vi "Configure Channels.vi"(8 "error in":errorcluster, 11 "Thermometer DAQmx RTD Cont CFG in":refnum<class "Thermometer DAQmx RTD Cont CFG.lvclass">) -> (0 "error out":errorcluster, 3 "Thermometer DAQmx RTD Cont CFG out":refnum<class "Thermometer DAQmx RTD Cont CFG.lvclass">)   [LabVIEW 2024, in "Thermometer DAQmx RTD Cont CFG.lvclass"]
uses:
  Thermometer DAQmx RTD Cont CFG.lvclass
  DAQmx Base CFG/DAQmx Base CFG.lvclass/DAQmx Base CFG.ctl
  Configurations/CFG Base/CFG Base.lvclass/CFG Base.ctl
  Thermometer DAQmx RTD Cont CFG.lvclass/Thermometer DAQmx RTD Cont CFG.ctl
  fbdc0025-8e19-453a-88be-6708611e45c6.vi
  fbdc0025-8e19-453a-88be-6708611e45c6.vi/a4169a97-72fc-4003-a778-603cf20cafa0.vi
  <vilib>/JDP Science/JSONtext/Find Item.vi
  <vilib>/JDP Science/JSONtext/Next JSON Value.vi
  <vilib>/JDP Science/JSONtext/String Subset.vi
  <vilib>/JDP Science/JSONtext/Parsing/Advance past next JSON Value (inlined COPY).vi
  <vilib>/JDP Science/JSONtext/Parsing/Advance past whitespace.vi
  <vilib>/JDP Science/JSONtext/Parsing/Advance past String.vi
  <vilib>/JDP Science/JSONtext/Parsing/Advance past Number.vi
  <vilib>/JDP Science/JSONtext/Parsing/Advance past Line Ending.vi
  <vilib>/JDP Science/JSONtext/Parsing/Parse Full Path or Item Name.vi
  <vilib>/JDP Science/JSONtext/Parsing/Advance past Array.vi
  <vilib>/JDP Science/JSONtext/Parsing/Advance past Object.vi
  <vilib>/JDP Science/JSONtext/support/Error Cluster From Code.vi
  <vilib>/JDP Science/JSONtext/Offset/Find Item Locations by Path.vi
  <vilib>/JDP Science/JSONtext/JSON text to Variant.vi
  <vilib>/Utility/error.llb/Error Cluster From Error Code.vi
  <vilib>/JDP Science/JSONtext/LVClass Serializer/JSONtext LVClass Serializer.lvclass
  <vilib>/DAQmx/create/channels.llb/DAQmx Create Channel (AI-Temperature-RTD).vi
  DAQmx Base CFG/DAQmx Base CFG.lvclass
  Configurations/CFG JSON/CFG JSON.lvclass
  Configurations/CFG Base/CFG Base.lvclass
  D:/git/HAL/HAL/Devices/DAQmx/DAQmx Base CFG/DAQmx Base CFG.lvclass
  D:/git/HAL/HAL/Configurations/CFG JSON/CFG JSON.lvclass
  D:/git/HAL/HAL/Configurations/CFG Base/CFG Base.lvclass
  D:/git/HAL/HAL/Devices/DAQmx/Thermo/Thermometer DAQmx RTD Cont CFG/Thermometer DAQmx RTD Cont CFG.lvclass
  Buffers/BufferLastReadingsDBL/BufferLastReadsDBL.lvclass
panel:
  out "units":i32(ring)=10143 items=["Deg C"=10143, "Deg F"=10144, "Kelvins"=10325, "Deg R"=10145, "From Custom Scale"=10065]
  out "rtd type":i32(ring)=12481 items=["Pt3750"=12481, "Pt3851"=10071, "Pt3911"=12482, "Pt3916"=10069, "Pt3920"=10053, "Pt3928"=12483, "Custom"=10137]
  out "current excitation source":i32(ring)=10167 items=["Internal"=10200, "External"=10167, "None"=10230]
  out "resistance cfg":i32(ring)=4 items=["2-Wire"=2, "3-Wire"=3, "4-Wire"=4]
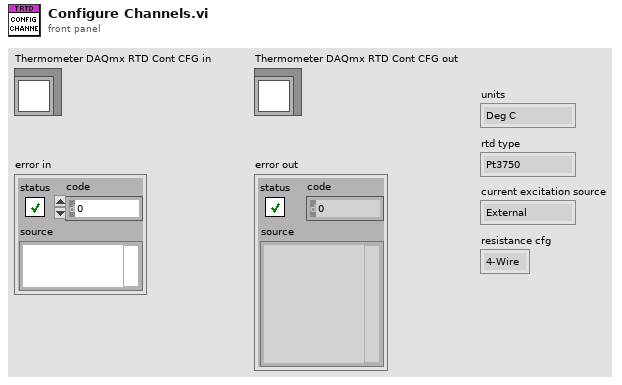
[diagram p1: front panel]
types:
  T1 = cluster{"Name":string, "Enabled":bool, "Minimum Value":dbl, "Maximum Value":dbl, "Resistance CFG":string, "R0":dbl, "Excitation Current":dbl, "Units":string, "Excitation Current Src":string, "RTD Type":string}[]
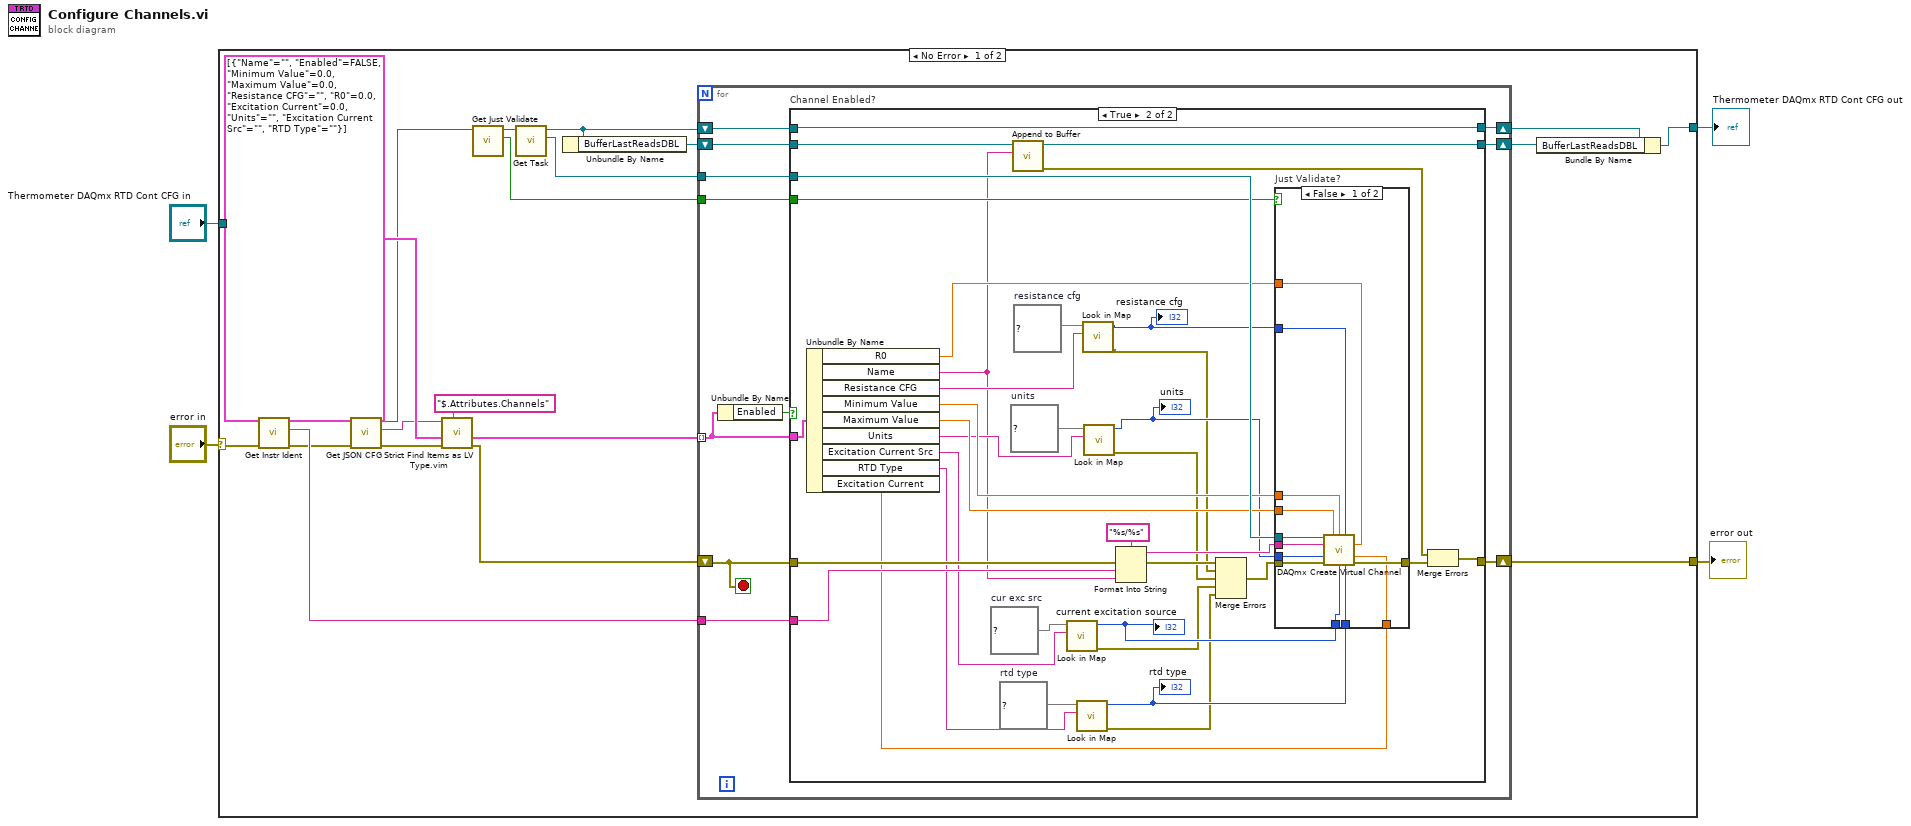
[diagram p0: block diagram]
diagram:
  n1 = case shown="No Error" "error in" {
    selector: "error in" -> [w19 w88]
    tunnel: "Thermometer DAQmx RTD Cont CFG in" -> [w15 w89]
    tunnel: [w20 w88] -> w1
    tunnel: [w7 w89] -> w2
    frame No Error {
      n2 = call-dynamic "Get Instr Ident.vi"("error in"=w19, "CFG JSON in"=w15) -> ("error out"=w11:errorcluster, "Instr Ident"=w21:string, "CFG JSON out"=w22:refnum<class "Thermometer DAQmx RTD Cont CFG.lvclass">)  [unwired: 7 in]
      n3 = call "Get JSON CFG.vi"("CFG JSON in"=w22) -> ("<JSON> CFG"=w18:string, "CFG JSON out"=w13:refnum<class "Thermometer DAQmx RTD Cont CFG.lvclass">)  [unwired: 9 in]
      n4 = call "Strict Find Items as LV Type.vim"("$Path or Item Name"="$.Attributes.Channels", "error in"=w11, "Data Type and Default Value"=T1 [{"Name"="", "Enabled"=FALSE, "Minimum Value"=0.0, "Maximum Value"=0.0, "Resistance CFG"="", "R0"=0.0, "Excitation Current"=0.0, "Units"="", "Excitation Current Src"="", "RTD Type"=""}], "<JSON>"=w18) -> ("error out"=w10:errorcluster, "Data out"=w16:T1)  [unwired: 5 in, 1 out]
      n5 = call "Get Just Validate.vi"("CFG Base in"=w13) -> ("Just Validate"=w14:bool, "CFG Base out"=w12:refnum<class "Thermometer DAQmx RTD Cont CFG.lvclass">)  [unwired: 9 in]
      n6 = call "Get Task.vi"("DAQmx Base CFG in"=w12) -> ("Task"=w17:refnum<k21>, "DAQmx Base CFG out"=w9:refnum<class "Thermometer DAQmx RTD Cont CFG.lvclass">)  [unwired: 9 in]
      n7 = Unbundle By Name(w9) -> ("BufferLastReadsDBL"=w8:refnum<class "BufferLastReadsDBL.lvclass">)
      n8 = for {
        tunnel: w16 -> [w32] mode=indexing
        shift-right: [w35] -> w20
        shift-left: w10 -> [w34]
        tunnel: w21 -> [w33]
        tunnel: w17 -> [w31]
        shift-right: [w30] -> w6
        shift-left: w9 -> [w29]
        tunnel: w14 -> [w27]
        shift-right: [w25] -> w5
        shift-left: w8 -> [w26]
        stop <- w34 stop-if-true
        n9 = Unbundle By Name(w32) -> ("Enabled"=w28:bool)
        n10 = case "Channel Enabled?" shown="True" w28 {
          tunnel: [w38 w40] -> w35
          tunnel: w34 -> [w38 w70]
          tunnel: w33 -> [_ w69]
          tunnel: w32 -> [_ w74]
          tunnel: [w37 w42] -> w30
          tunnel: w31 -> [_ w72]
          tunnel: w29 -> [w37 w42]
          tunnel: w27 -> [_ w65]
          tunnel: w26 -> [w36 w44]
          tunnel: [w36 w41] -> w25
          frame False {
          }
          frame True {
            w48 = map{string, i32} {"2-Wire"=2, "3-Wire"=3, "4-Wire"=4}  # resistance cfg
            w53 = map{string, i32} {"External"=10167, "Internal"=10200, "None"=10230}  # cur exc src
            w56 = map{string, i32} {"Custom"=10137, "Pt3750"=12481, "Pt3851"=10071, "Pt3911"=12482, "Pt3916"=10069, "Pt3920"=10053, "Pt3928"=12483}  # rtd type
            w60 = map{string, i32} {"Deg C"=10143, "Deg F"=10144, "Deg R"=10145, "From Custom Scale"=10065, "Kelvins"=10325}  # units
            n11 = Unbundle By Name(w74) -> ("R0"=w64:dbl, "Name"=w43:string, "Resistance CFG"=w47:string, "Minimum Value"=w63:dbl, "Maximum Value"=w62:dbl, "Units"=w58:string, "Excitation Current Src"=w52:string, "RTD Type"=w55:string, "Excitation Current"=w61:dbl)
            n12 = call "Append to Buffer.vi"("Channel"=w43, "BufferLastReadingsDBL in"=w44) -> ("error out"=w39:errorcluster, "BufferLastReadingsDBL out"=w41:refnum<class "BufferLastReadsDBL.lvclass">)  [unwired: 8 in]
            n13 = call "Look in Map.vi"("Key"=w52, "Map"=w53) -> ("error out"=w49:errorcluster, "Value"=w51:i32)  [unwired: 8 in]
            "current excitation source" <- w51
            n14 = call "Look in Map.vi"("Key"=w55, "Map"=w56) -> ("error out"=w50:errorcluster, "Value"=w54:i32)  [unwired: 8 in]
            "rtd type" <- w54
            n15 = call "Look in Map.vi"("Key"=w47, "Map"=w48) -> ("error out"=w45:errorcluster, "Value"=w46:i32)  [unwired: 8 in]
            "resistance cfg" <- w46
            n16 = call "Look in Map.vi"("Key"=w58, "Map"=w60) -> ("error out"=w57:errorcluster, "Value"=w59:i32)  [unwired: 8 in]
            "units" <- w59
            n17 = Format Into String(format string="%s/%s", error in=w70, w69, w43) -> (resulting string=w67:string, error out=w68:errorcluster)  [unwired: 1 in]
            n18 = Merge Errors(w68, w45, w57, w49, w50) -> (w66:errorcluster)
            n19 = case "Just Validate?" shown="False" w65 {
              tunnel: w66 -> [w86 w87]
              tunnel: w67 -> [w83 _]
              tunnel: w72 -> [w85 _]
              tunnel: [w84 w87] -> w73
              tunnel: w46 -> [w82 _]
              tunnel: w64 -> [w81 _]
              tunnel: w63 -> [w80 _]
              tunnel: w62 -> [w79 _]
              tunnel: w59 -> [w78 _]
              tunnel: w54 -> [w77 _]
              tunnel: w51 -> [w76 _]
              tunnel: w61 -> [w75 _]
              frame False {
                n20 = call-poly <vilib>:"DAQmx Create Virtual Channel.vi"("task in"=w85, "maximum value"=w79, "minimum value"=w80, "resistance configuration"=w82, "physical channels"=w83, "r0"=w81, "units"=w78, "current excitation value"=w75, "error in"=w86, "current excitation source"=w76, "rtd type"=w77) -> ("error out"=w84:errorcluster)  [unwired: 3 in, 1 out]
              }
              frame True {
              }
            }
            n21 = Merge Errors(w39, w73) -> (w40:errorcluster)
          }
        }
      }
      n22 = Bundle By Name(cluster=w6, "BufferLastReadsDBL"=w5) -> (w7:refnum<class "Thermometer DAQmx RTD Cont CFG.lvclass">)
    }
    frame Error {
    }
  }
  "error out" <- w1
  "Thermometer DAQmx RTD Cont CFG out" <- w2
